vi "Do.vi"(8 "error in (no error)":errorcluster, 10 "Actor in":refnum<class "Actor.lvclass">, 11 "Hold Msg":refnum<class "Hold Msg.lvclass">) -> (0 "error out":errorcluster, 2 "Actor out":refnum<class "Actor.lvclass">)   [LabVIEW 2020, in "PS Control Actor.lvlib" / "Hold Msg.lvclass"]
doc: "This VI delivers the message to the actor by calling the appropriate method(s) on the actor."
uses:
  Hold Msg.lvclass
  <vilib>/ActorFramework/Actor/Actor.lvclass
  PS Control Actor/PS Control Actor.lvclass
  Applications/National Instruments/LabVIEW 2020 64-bit/vi.lib/ActorFramework/Actor/Actor.lvclass
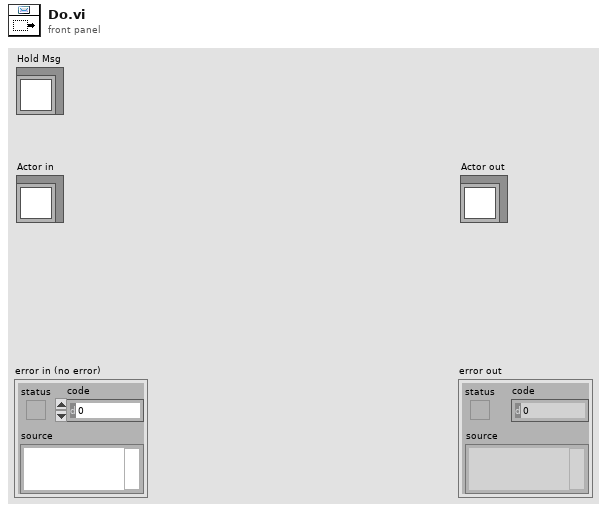
[diagram p1: front panel]
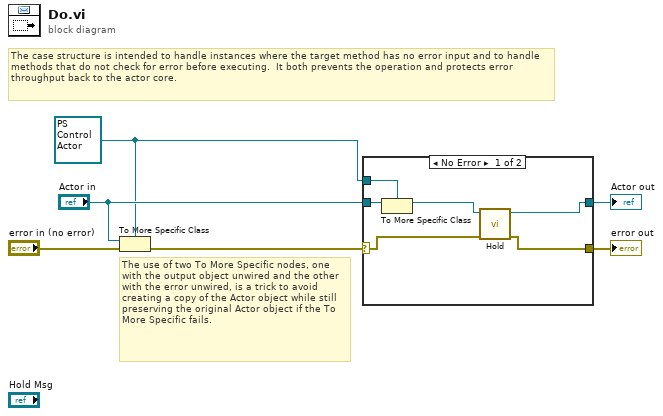
[diagram p0: block diagram]
diagram:
  w1 = refnum<class "PS Control Actor.lvclass"> refnum ("Actor in")
  # "The use of two To More Specific nodes, one with the output object unwired and the other with the error unwired, is a trick to avoid creating a copy of the Actor object while still preserving the original Actor object if the To More Specific fails."
  # "The case structure is intended to handle instances where the target method has no error input and to handle methods that do not check for error before executing.  It both prevents the operation and protects error throughput back to the actor core."
  n1 = To More Specific Class(target class=w1, reference="Actor in", error in="error in (no error)") -> (error out=w5:errorcluster)  [unwired: 1 out]
  n2 = case shown="No Error" w5 {
    selector: w5 -> [w9 w14]
    tunnel: [w8 w14] -> w4
    tunnel: [w7 w13] -> w3
    tunnel: "Actor in" -> [w12 w13]
    tunnel: w1 -> [w11 _]
    frame No Error {
      n3 = To More Specific Class(target class=w11, reference=w12) -> (specific class reference=w10:refnum<class "PS Control Actor.lvclass">)  [unwired: 1 in, 1 out]
      n4 = call-dynamic "Hold.vi"("error in (no error)"=w9, "PS Control Actor in"=w10) -> ("error out"=w8:errorcluster, "PS Control Actor out"=w7:refnum<class "PS Control Actor.lvclass">)  [unwired: 8 in]
    }
    frame Error {
      # "If type check fails, pass the original object out again."
    }
  }
  "error out" <- w4
  "Actor out" <- w3
